vi "判断设备归属地.vi"(10 "待查询设备MAC":string=" ", 11 "个人剂量仪-云服务器.i":refnum<class "个人剂量仪-云服务器.lvclass">) -> (1 "找到匹配？":bool, 3 "匹配的企业":string, 4 "所有企业名":string[](array[string]))   [LabVIEW 2013, in "个人剂量仪-云服务器.lvclass"]
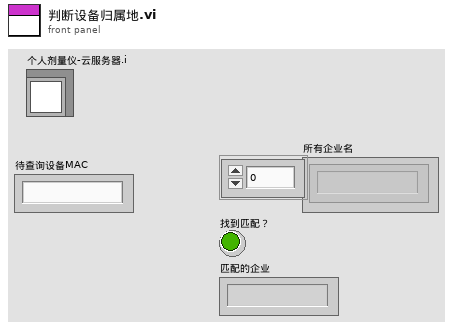
[diagram p1: front panel]
types:
  T1 = cluster{"企业信息":cluster{"登录名":string, "密码":string, "企业名称":string, "邮箱":string, "电话":string}, "用户列表":cluster{"用户名":string, "设备MAC":string, "设备状态":i32, "密码":string, "职类":i32, "姓名":string, "电话":string, "邮箱":string, "备注":string, "最后活动":string}[]}[]
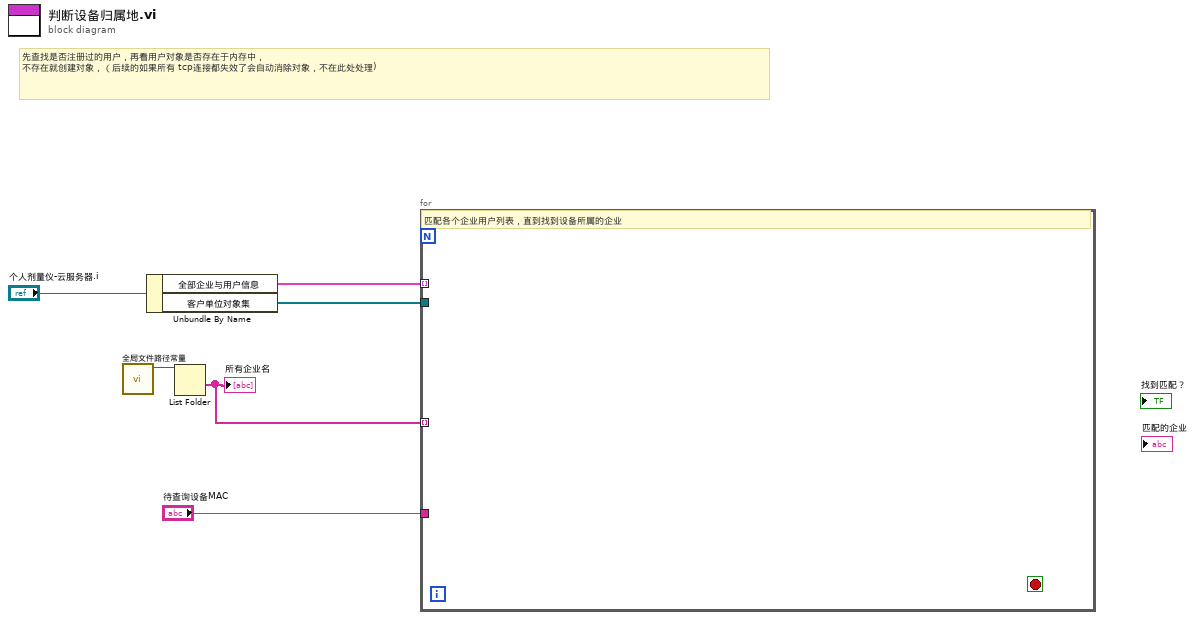
[diagram p0: block diagram]
diagram:
  # "先查找是否注册过的用户，再看用户对象是否存在于内存中，\n不存在就创建对象，（后续的如果所有 tcp连接都失效了会自动消除对象，不在此处处理)"
  n1 = call "全局文件路径常量.vi"() -> ("用户数据库根目录"=w6:path)  [unwired: 9 in, 2 out]
  n2 = Unbundle By Name("个人剂量仪-云服务器.i") -> ("全部企业与用户信息"=w2:T1, "客户单位对象集"=w1:refnum<class "客户单位.lvclass">[])
  n3 = List Folder(path=w6) -> (folder names=w5:string[])  [unwired: 3 in, 3 out]
  "所有企业名" <- w5
  n4 = for {
    tunnel: w5 -> [_] mode=indexing
    tunnel: "待查询设备MAC" -> [_]
    tunnel: w2 -> [_] mode=indexing
    tunnel: w1 -> [_]
    stop <- _ stop-if-true
    # "匹配各个企业用户列表，直到找到设备所属的企业"
  }
